vi "Pre Launch Init.vi"(11 "Test_Nested in":refnum<class "Test_Nested.lvclass">) -> (0 "error out":errorcluster, 3 "Test_Nested out":refnum<class "Test_Nested.lvclass">)   [LabVIEW 2025, in "Test_Nested.lvlib" / "Test_Nested.lvclass"]
doc: "<p>(<strong>Filename</strong>: <span class=\"dnl\">Actor Framework.lvlib:Actor.lvclass:Pre Launch Init.vi</span>)</p>\n<p>Defines behavior that occurs after the <a href=\"nihelplauncher://docs/csh?context=lvcore_lvcomm_af_launch_nested_actor\">Launch Nested Actor</a> method is invoked but before the actor's Actor Core method begins running.</p>\n<p>By default, this method does nothing. A descendant class may override it to define behavior.</p>"
uses:
  Test_Nested.lvclass
  Test_Nested.lvclass/Test_Nested.ctl
  <vilib>/ActorFramework/Actor/Actor.lvclass
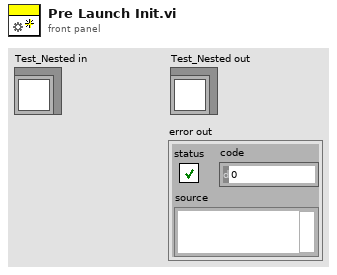
[diagram p1: front panel]
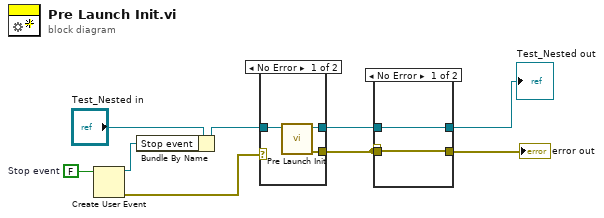
[diagram p0: block diagram]
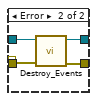
[diagram p2: hidden frame]
diagram:
  w7 = FALSE  # Stop event
  n1 = Create User Event(user event datatype=w7) -> (user event=w5:refnum<user-event>, error out=w4:errorcluster)  [unwired: 1 in]
  n2 = Bundle By Name(cluster="Test_Nested in", "Stop event"=w5) -> (w6:refnum<class "Test_Nested.lvclass">)
  n3 = case shown="No Error" w4 {
    selector: w4 -> [_ w13]
    tunnel: [w12 w13] -> w1
    tunnel: [w11 w14] -> w9
    tunnel: w6 -> [w10 w14]
    frame No Error {
      n4 = call-parent "Pre Launch Init.vi"("Actor in"=w10) -> ("error out"=w12:errorcluster, "Actor out"=w11:refnum<class "Test_Nested.lvclass">)  [unwired: 9 in]
    }
    frame Error {
    }
  }
  n5 = case shown="No Error" w1 {
    selector: w1 -> [w16 w17]
    tunnel: w9 -> [w15 w20]
    tunnel: [w15 w19] -> w3
    tunnel: w1 -> [_ _]
    tunnel: [w16 w18] -> w2
    frame No Error {
    }
    frame Error {
      n6 = call-dynamic "Destroy_Events.vi"("error in (no error)"=w17, "Test_Nested in"=w20) -> ("error out"=w18:errorcluster, "Test_Nested out"=w19:refnum<class "Test_Nested.lvclass">)  [unwired: 8 in]
    }
  }
  "error out" <- w2
  "Test_Nested out" <- w3
